vi "AutoEnumToString.vi"(10 "AutoEnum":T1) -> (2 "EnumString":string)   [LabVIEW 2012]
uses:
  AutoEnum.ctl
  Sally_Dashboard_2013/DBNameEnum.ctl
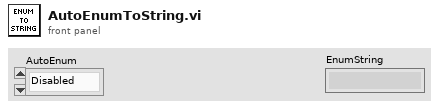
[diagram p1: front panel]
types:
  T1 = typedef "AutoEnum.ctl" = enum16{"Disabled", "BackRight", "BackLeft", "CloseRight", "CloseLeft", "BehindPyramid"}
  T2 = typedef "DBNameEnum.ctl" = enum16{"AutoEnum", "DriveLoopTime", "DriveAlignLS", "ClimbLS", "LauncherAngleMatches", "FrameworkVersion", "sLauncherAngle", "LauncherTargetAngle", "sLauncherRPM", "LauncherTargetRPM", "sDriveDistance", "LauncherMotorValue", "PullbackTol", "FireTol", "LauncherRPMTol", "LauncherAngleTol", "BackRight", "CloseLeft", "BehindPyramid", "Disabled", "CloseRight", "BackLeft", "InitialWait", "WaitBetweenLaunch", "AngleCluster", "RPMCluster", "UseAngleEncoder", "UseLauncherEncoder", "UseLauncherPID"}
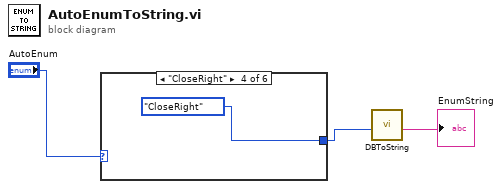
[diagram p0: block diagram]
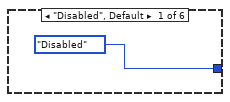
[diagram p2: hidden frame]
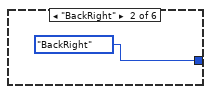
[diagram p3: hidden frame]
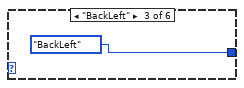
[diagram p4: hidden frame]
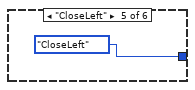
[diagram p5: hidden frame]
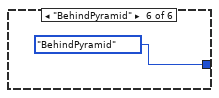
[diagram p6: hidden frame]
diagram:
  n1 = case shown="\"CloseRight\"" "AutoEnum" {
    tunnel: [DBNameEnum."Disabled" ("Enum") DBNameEnum."BackRight" ("Enum") DBNameEnum."BackLeft" ("Enum") DBNameEnum."CloseRight" ("Enum") DBNameEnum."CloseLeft" ("Enum") DBNameEnum."BehindPyramid" ("Enum")] -> w2
    frame "Disabled", Default {
    }
    frame "BackRight" {
    }
    frame "BackLeft" {
    }
    frame "CloseRight" {
    }
    frame "CloseLeft" {
    }
    frame "BehindPyramid" {
    }
  }
  n2 = call "DBToString.vi"("Enum"=w2) -> ("Refname"=→"EnumString":string)  [unwired: 9 in]
